vi "XLS_to_TXT.vi"(8 "error in (no error)":errorcluster, 11 "Path":path) -> (0 "error out":errorcluster, 3 "Path out":path=path "c:/temp/setup-temp.txt")   [LabVIEW 2011]
panel:
  in  "Excel._Application":refnum<k7>
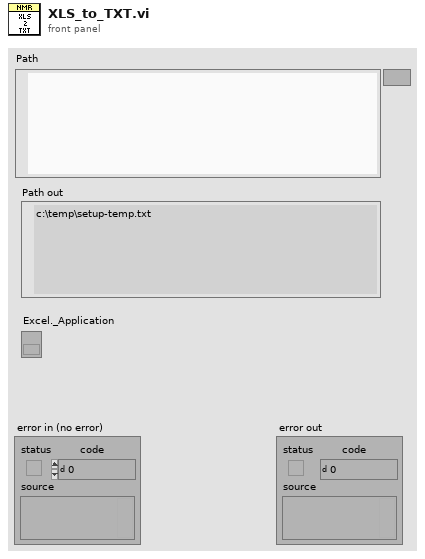
[diagram p1: front panel]
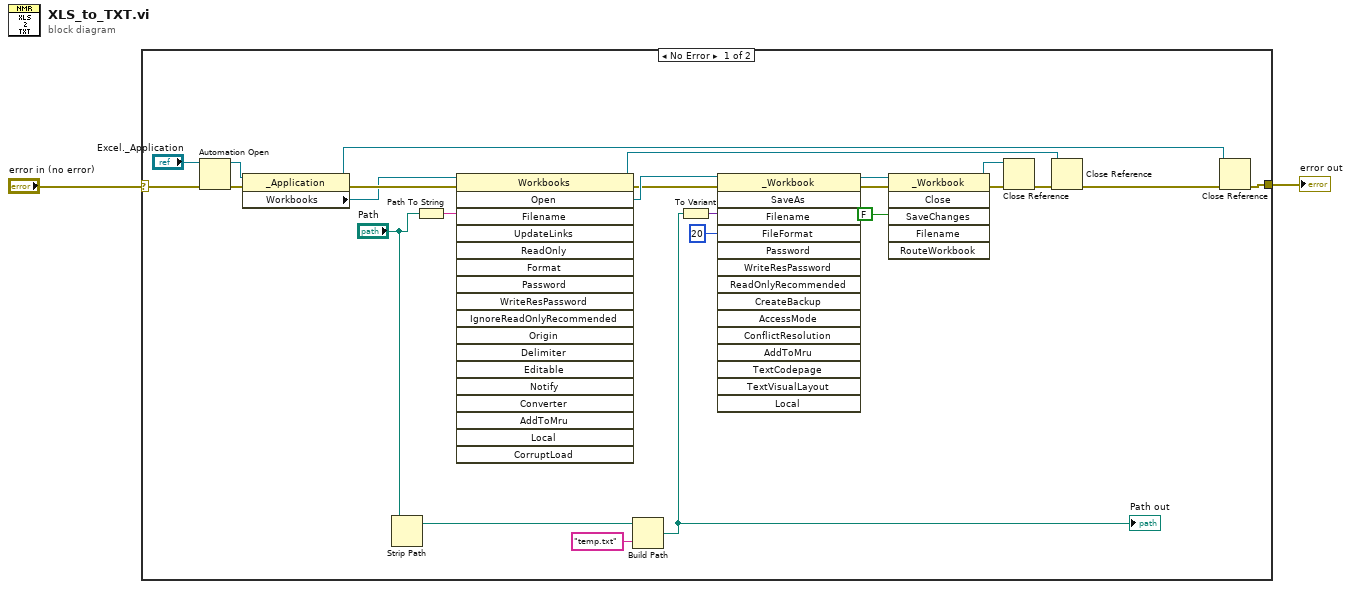
[diagram p0: block diagram]
diagram:
  n1 = case shown="No Error" "error in (no error)" {
    selector: "error in (no error)" -> [w16 w27]
    tunnel: [w13 w27] -> w2
    frame No Error {
      n2 = Automation Open(error in (no error)=w16, Automation Refnum="Excel._Application") -> (Automation Refnum=w25:refnum<k7>, error out=w24:errorcluster)  [unwired: 2 in]
      n3 = property class="_Application"(reference=w25, error in=w24) -> (reference out=w8:refnum<k7>, error out=w23:errorcluster, "Workbooks"=w18:refnum<k7>)
      n4 = Strip Path(path="Path") -> (stripped path=w6:path)  [unwired: 1 out]
      n5 = Path To String(path="Path") -> (string=w17:string)
      n6 = invoke class="Workbooks" method="Open"(reference=w18, error in=w23, "Filename"=w17) -> (reference out=w15:refnum<k7>, error out=w21:errorcluster, "Open"=w22:refnum<k7>)  [unwired: 15 in, 15 out]
      n7 = Build Path(base path=w6, name or relative path="temp.txt") -> (appended path=w4:path)
      "Path out" <- w4
      n8 = To Variant(anything=w4) -> (Variant=w19:variant)
      n9 = invoke class="_Workbook" method="SaveAs"(reference=w22, error in=w21, "Filename"=w19, "FileFormat"=20) -> (reference out=w12:refnum<k7>, error out=w20:errorcluster)  [unwired: 11 in, 13 out]
      n10 = invoke class="_Workbook" method="Close"(reference=w12, "SaveChanges"=FALSE) -> (reference out=w11:refnum<k7>)  [unwired: 4 in, 5 out]
      n11 = Close Reference(reference=w11, error in (no error)=w20) -> (error out=w14:errorcluster)
      n12 = Close Reference(reference=w15, error in (no error)=w14) -> (error out=w9:errorcluster)
      n13 = Close Reference(reference=w8, error in (no error)=w9) -> (error out=w13:errorcluster)
    }
    frame Error {
    }
  }
  "error out" <- w2
